vi "例题7.1.vi"() -> ()   [LabVIEW 2017]
panel:
  out "7（X0=10，dx=2，Y）多条曲线":cluster{i32, i32, cluster{dbl[]}[]}(graph)
  out "6（X0=10，dx=2，Y）多条曲线":cluster{i32, i32, dbl[][]}(graph)
  out "5（X0=10，dx=2，Y）多条曲线":cluster{i32, i32, dbl[]}[](graph)
  out "4（X0=10，dx=2，Y）单条曲线":cluster{i32, i32, dbl[]}(graph)
  out "3（Y）多条曲线":cluster{dbl[]}[](graph)
  out "2（Y）多条曲线":dbl[][](graph)
  out "1(Y)单条曲线":dbl[](graph)
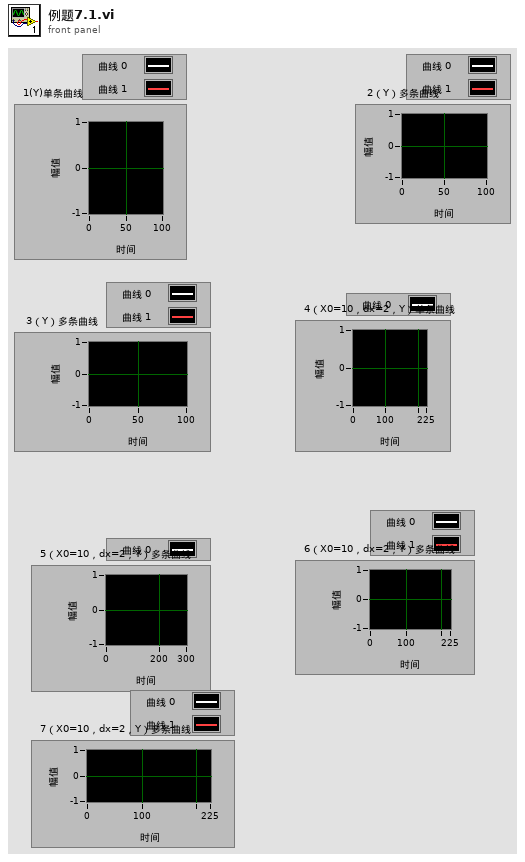
[diagram p1: front panel]
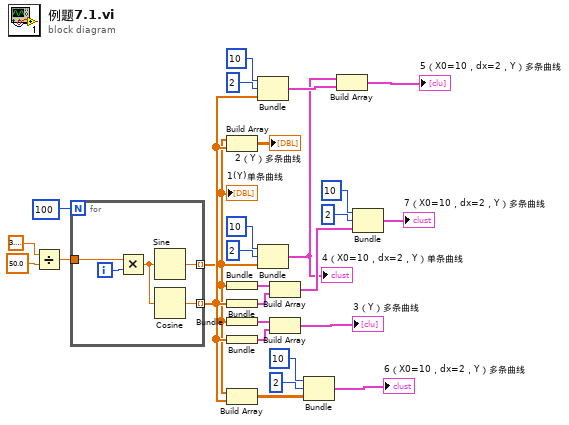
[diagram p0: block diagram]
diagram:
  n1 = Divide(x=3.141592653589793, y=50.0) -> (x/y=w25:dbl)
  n2 = for {
    N: 100 -> [_]
    tunnel: w25 -> [w32]
    tunnel: [w29] -> w4 mode=indexing
    tunnel: [w28] -> w5 mode=indexing
    i -> [w31]
    n3 = Multiply(x=w32, y=w31) -> (x*y=w30:dbl)
    n4 = Sine(x=w30) -> (sin(x)=w29:dbl)
    n5 = Cosine(x=w30) -> (cos(x)=w28:dbl)
  }
  "1(Y)单条曲线" <- w4
  n6 = Build Array(w4, w5) -> (→"2（Y）多条曲线":dbl[][])
  n7 = Bundle(w4) -> (w3:cluster{dbl[]})  [unwired: 1 in]
  n8 = Bundle(w5) -> (w2:cluster{dbl[]})  [unwired: 1 in]
  n9 = Bundle(w4) -> (w22:cluster{dbl[]})  [unwired: 1 in]
  n10 = Bundle(w5) -> (w21:cluster{dbl[]})  [unwired: 1 in]
  n11 = Build Array(w4, w5) -> (w14:dbl[][])
  n12 = Bundle(10, 2, w5) -> (w15:cluster{i32, i32, dbl[]})  [unwired: 1 in]
  n13 = Bundle(10, 2, w4) -> (w8:cluster{i32, i32, dbl[]})  [unwired: 1 in]
  "4（X0=10，dx=2，Y）单条曲线" <- w8
  n14 = Build Array(w3, w2) -> (w11:cluster{dbl[]}[])
  n15 = Build Array(w22, w21) -> (→"3（Y）多条曲线":cluster{dbl[]}[])
  n16 = Bundle(10, 2, w14) -> (→"6（X0=10，dx=2，Y）多条曲线":cluster{i32, i32, dbl[][]})  [unwired: 1 in]
  n17 = Build Array(w8, w15) -> (→"5（X0=10，dx=2，Y）多条曲线":cluster{i32, i32, dbl[]}[])
  n18 = Bundle(10, 2, w11) -> (→"7（X0=10，dx=2，Y）多条曲线":cluster{i32, i32, cluster{dbl[]}[]})  [unwired: 1 in]
